vi "F Dwf Analog Out Symmetry Info.vi"(7 "ppercentageMax":dbl, 8 "error in (no error)":errorcluster, 9 "ppercentageMin":dbl, 10 "idxChannel":i32, 11 "hdwf":i32) -> (0 "error out":errorcluster, 1 "ppercentageMin out":dbl, 3 "function return":i32, 5 "ppercentageMax out":dbl)   [LabVIEW 2019, in "Olasdwf.lvlib"]
doc: "DWFAPI int FDwfAnalogOutSymmetryInfo(HDWF hdwf, int idxChannel, double *ppercentageMin, double *ppercentageMax);"
uses:
  Olasdwf.lvlib
  Windows/System32/dwf.dll
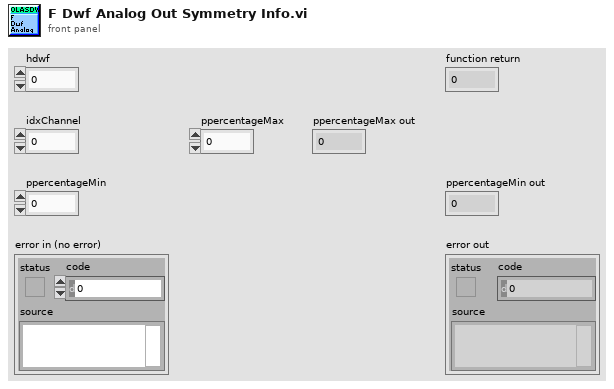
[diagram p1: front panel]
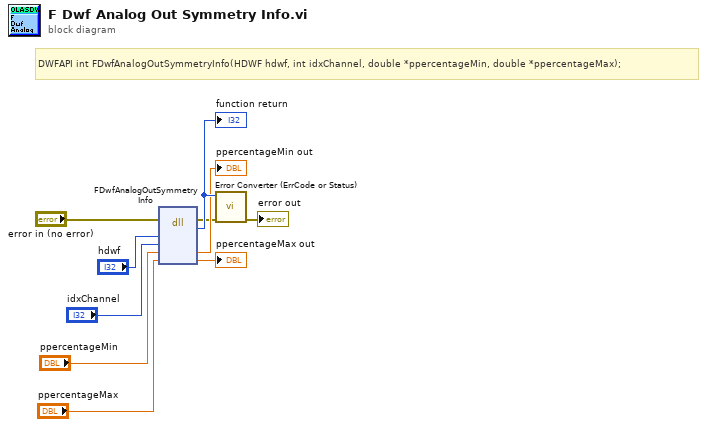
[diagram p0: block diagram]
diagram:
  # "DWFAPI int FDwfAnalogOutSymmetryInfo(HDWF hdwf, int idxChannel, double *ppercentageMin, double *ppercentageMax);"
  n1 = dll-call lib="C:/Windows/System32/dwf.*" fn="FDwfAnalogOutSymmetryInfo"(error in="error in (no error)", "hdwf"="hdwf", "idxChannel"="idxChannel", "ppercentageMin"="ppercentageMin", "ppercentageMax"="ppercentageMax") -> (error out=w2:errorcluster, w10:i32, "ppercentageMin"=→"ppercentageMin out":dbl, "ppercentageMax"=→"ppercentageMax out":dbl)  [unwired: 4 in, 1 out]
  "function return" <- w10
  n2 = call "Error Converter (ErrCode or Status).vi"("error in (no error)"=w2, "error code"=w10) -> ("error out"=→"error out":errorcluster)  [unwired: 9 in]
